vi "uTTA_Calibration_VOffs.vi"(6 "AR488_in":refnum<visa-resource-name>, 7 "CommandQueue":refnum<queue>, 8 "error in":errorcluster, 9 "FunctionGen":refnum<visa-resource-name>, 10 "DataQueue":refnum<queue>, 11 "FDMS_FileIn":refnum<k34>) -> (0 "error out":errorcluster, 1 "FunctionGen_out":refnum<visa-resource-name>, 2 "abort":bool, 3 "FDMS_FileOut":refnum<k34>, 4 "AR488_out":refnum<visa-resource-name>)   [LabVIEW 2021]
uses:
  <vilib>/Utility/miscctls.llb/LVPointTypeDef.ctl
  <vilib>/Analysis/6fits.llb/Curve Fitting Criteria.ctl
  98f5d860-8e0d-4648-8282-1f02ee17b982.vi
  <vilib>/Analysis/NI_AALPro.lvlib
panel:
  out "Channel":i32
  out "VOFF Cal.":T1(graph)
  out "VOFF DAC slope":dbl format="%#_4pV/Digit"
  out "VOFF DAC Residue":dbl caption="Residue" format="%.3p"
  out "VOFF DAC Offset":dbl format="%#_6pV"
  out "ADC_Values":dbl[](array[numeric]) format="%#.2g"
  out "ADC_Variance":dbl[](array[numeric]) format="%#.2g"
  in  "Start DAC VOFF":bool
  in  "VOFF DAC Inc":i32=1000 caption="DAC Incements" min=0 max=32767 step=1 format="%d Counts/Step"
  out "Status":string="Exit"
  in  "stop":bool
  # "1. Connect the DMM in voltage measurement mode between the TP323.x and Ground \n2. Connect a ground lead to the outer Conductor of the BNC line to provide propper grounding\n3. Start the calibration"
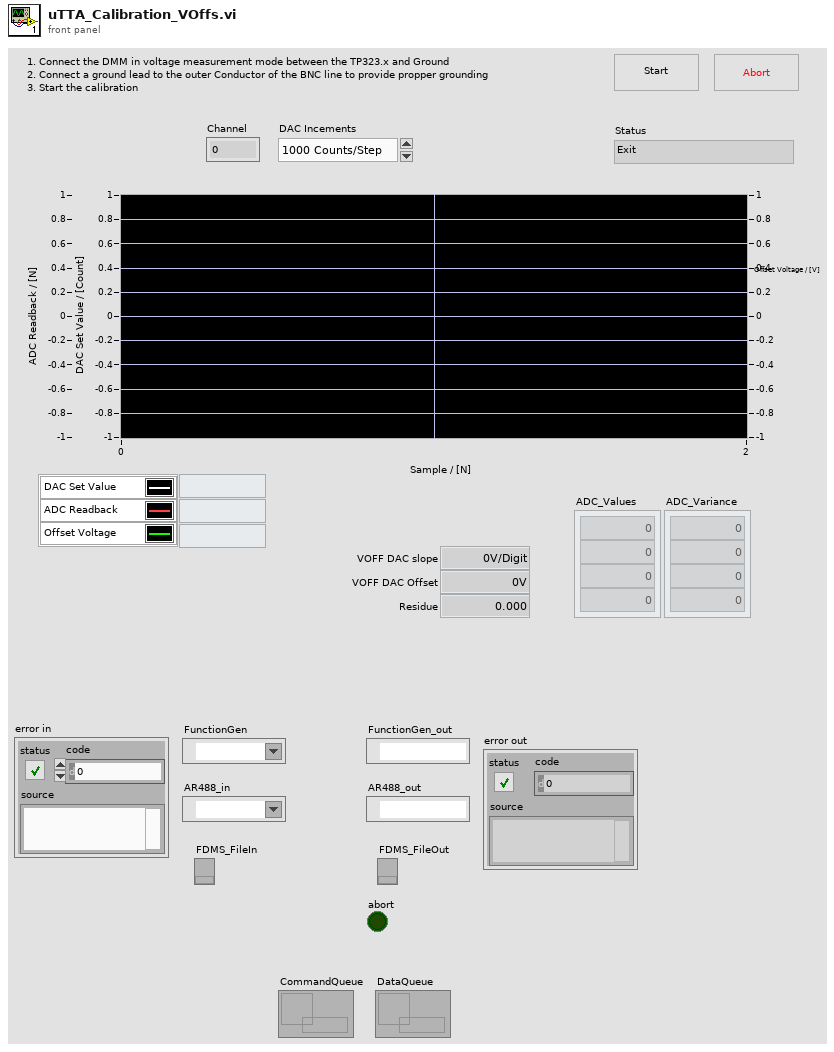
[diagram p1: front panel]
types:
  T1 = cluster{"Ref_Voltage":dbl, "mean":dbl, "mean":dbl}
  T2 = typedef "LVPointTypeDef.ctl" = cluster{"Horizontal":i16, "Vertical":i16}
  T3 = cluster{"Ref_Voltage":dbl, "mean":dbl, "mean":dbl}[]
  T4 = typedef "NI_AALPro.lvlib/Curve Fitting Criteria.ctl" = u16
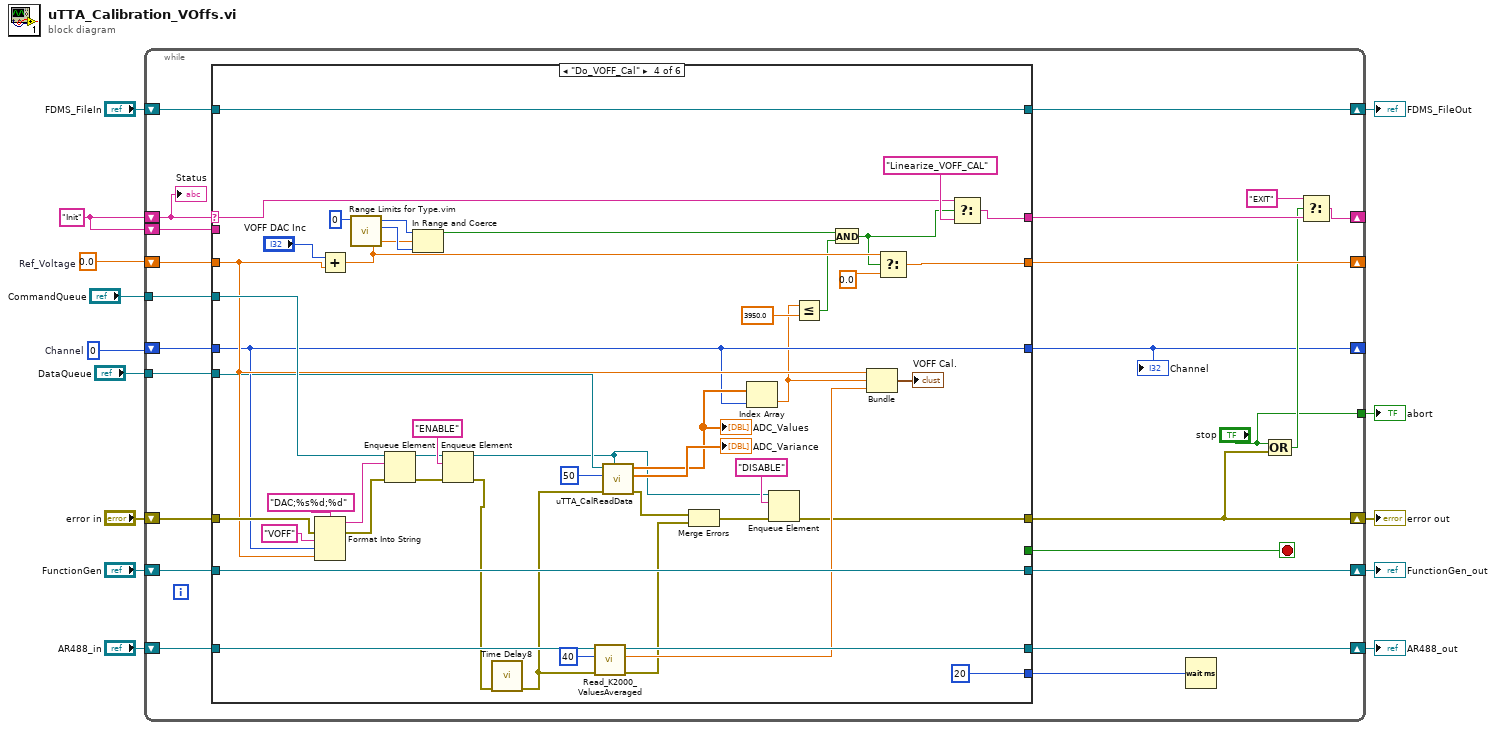
[diagram p0: block diagram]
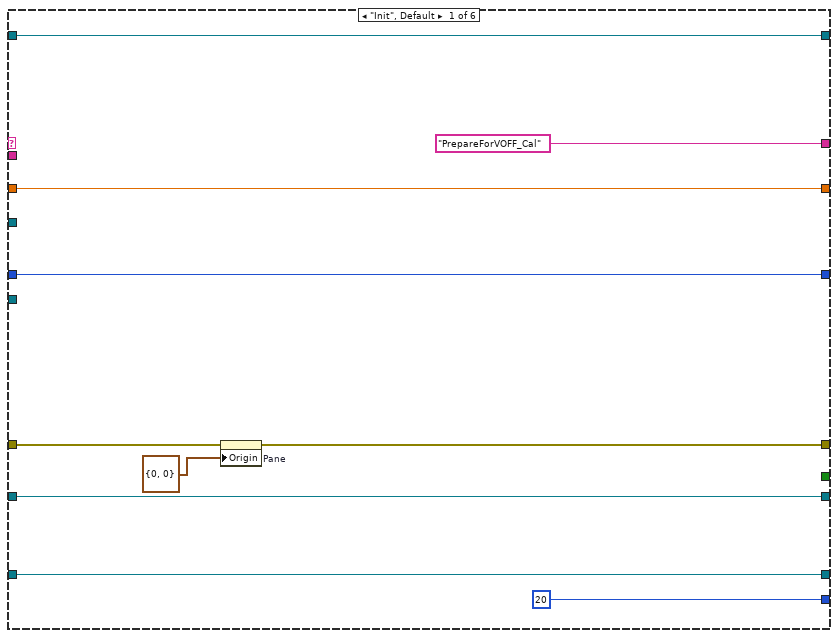
[diagram p2: hidden frame]
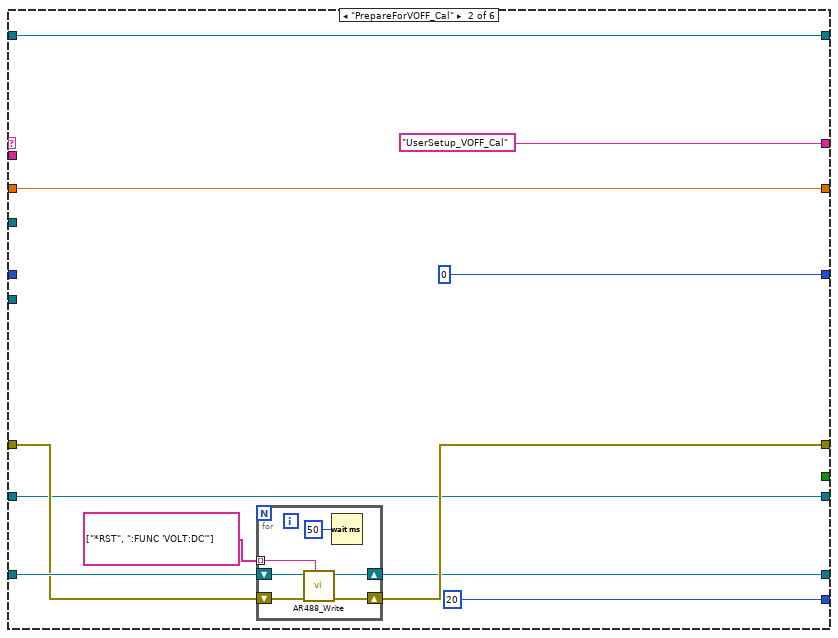
[diagram p3: hidden frame]
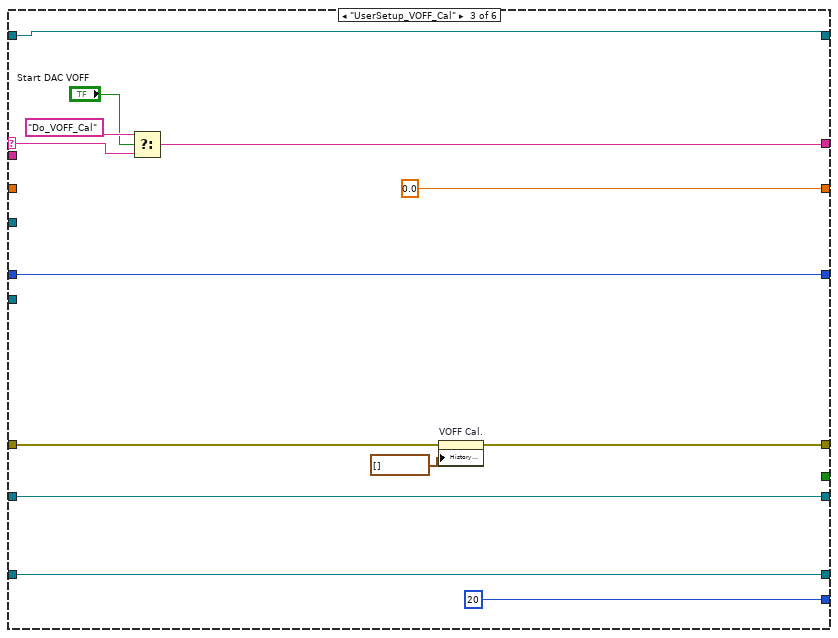
[diagram p4: hidden frame]
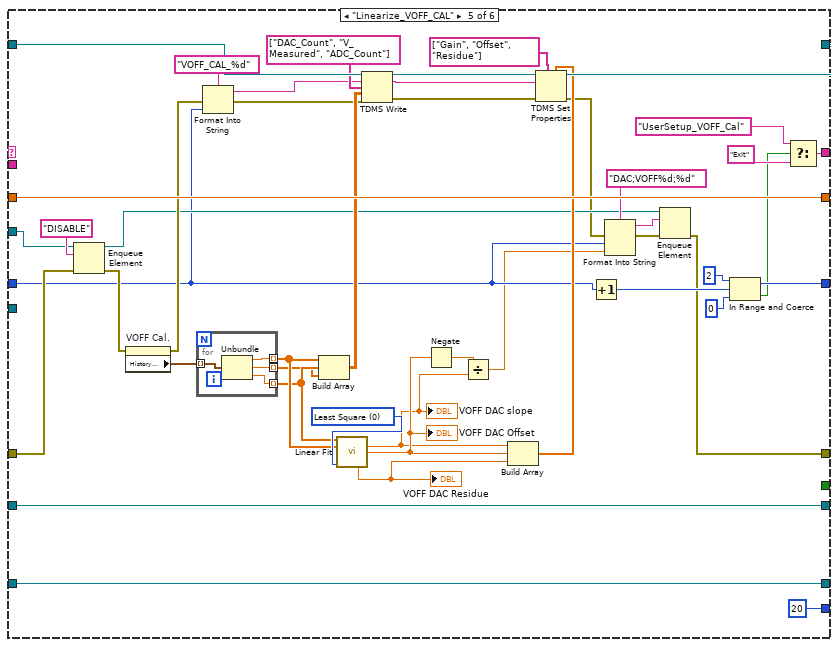
[diagram p5: hidden frame]
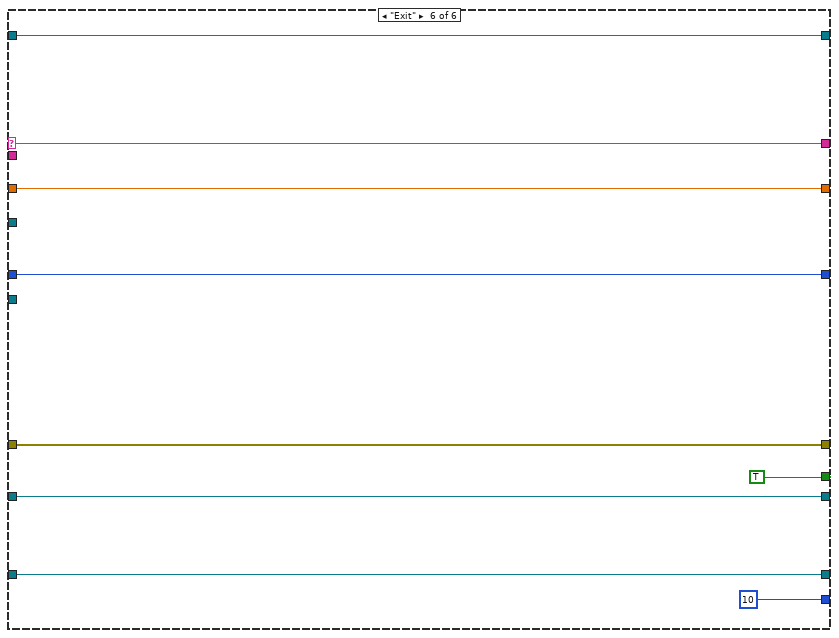
[diagram p6: hidden frame]
diagram:
  w12 = 0  # Channel
  w14 = 0.0  # Ref_Voltage
  w13 = "Init"
  n1 = while {
    shift-right: [w24] -> _
    shift-left: w13 -> [w35]
    shift-right: [w22] -> w7
    shift-left: "error in" -> [w37]
    shift-right: [w33] -> w8
    shift-left: "FunctionGen" -> [w34]
    shift-right: [w32] -> w9
    shift-left: "AR488_in" -> [w31]
    shift-left: w13 -> [w30]
    tunnel: "CommandQueue" -> [w29]
    tunnel: "DataQueue" -> [w28]
    shift-right: [w26] -> _
    shift-left: w14 -> [w27]
    shift-right: [w19] -> w2
    shift-left: "FDMS_FileIn" -> [w18]
    shift-right: [w16] -> _
    shift-left: w12 -> [w17]
    tunnel: ["stop"] -> w1
    stop <- w20 stop-if-true
    n2 = case shown="\"Do_VOFF_Cal\"" w35 {
      selector: w35 -> [_ _ w70 w102 _ w182]
      tunnel: [_ _ _ _ _ TRUE] -> w20
      tunnel: w37 -> [w44 w50 w66 w117 w137 w176]
      tunnel: ["PrepareForVOFF_Cal" ("t") "UserSetup_VOFF_Cal" ("t") w69 w105 w161 w182] -> w25
      tunnel: [w40 w54 w65 w78 w125 w176] -> w22
      tunnel: [u32 20 u32 20 u32 20 u32 20 u32 20 u32 10] -> w36
      tunnel: w34 -> [w43 w49 w77 w123 w169 w175]
      tunnel: [w43 w49 w77 w123 w169 w175] -> w33
      tunnel: [w42 w53 w76 w107 w168 w174] -> w32
      tunnel: w31 -> [w42 w52 w76 w106 w168 w174]
      tunnel: w30 -> [_ _ _ _ _ _]
      tunnel: w29 -> [_ _ _ w121 w138 _]
      tunnel: w28 -> [_ _ _ w93 _ _]
      tunnel: w27 -> [w41 w57 _ w99 w167 w178]
      tunnel: [w41 w57 0.0 w111 w167 w178] -> w26
      tunnel: [w39 w51 w72 w122 w152 w179] -> w19
      tunnel: w18 -> [w39 w51 w72 w122 w151 w179]
      tunnel: w17 -> [w38 _ w71 w95 w128 w177]
      tunnel: [w38 0 ("Channel") w71 w95 w162 w177] -> w16
      frame "Init", Default {
        n3 = property on="Pane" class="Pane"(error in=w44, "Origin"=T2 {"Horizontal"=0, "Vertical"=0}) -> (error out=w40:errorcluster)  [unwired: 1 in, 1 out]
      }
      frame "PrepareForVOFF_Cal" {
        n4 = for {
          tunnel: string[] ["*RST", ":FUNC 'VOLT:DC'"] -> [w63] mode=indexing
          shift-right: [w61] -> w53
          shift-left: w52 -> [w64]
          shift-right: [w60] -> w54
          shift-left: w50 -> [w62]
          n5 = call "AR488_Write.vi"("write"=w63, "error in (no error)"=w62, "VISA Refnum in"=w64) -> ("error out"=w60:errorcluster, "VISA Refnum out"=w61:refnum<visa-resource-name>)  [unwired: 7 in]
          n6 = Wait (ms)(milliseconds to wait=u32 50) -> ()  [unwired: 1 out]
        }
      }
      frame "UserSetup_VOFF_Cal" {
        n7 = Select(t="Do_VOFF_Cal", s="Start DAC VOFF", f=w70) -> (s? t:f=w69:string)
        n8 = property on="VOFF Cal." class="WFChart (strict)"(error in=w66, "History Data"=T3 []) -> (error out=w65:errorcluster)  [unwired: 1 in, 1 out]
      }
      frame "Do_VOFF_Cal" {
        n9 = Format Into String(format string="DAC;%s%d;%d" ("element"), error in=w117, "VOFF" ("input 1"), w95, w99) -> (resulting string=w119:string, error out=w116:errorcluster)  [unwired: 1 in]
        n10 = Add(x="VOFF DAC Inc", y=w99) -> (x+y=w101:dbl)
        n11 = call "Range Limits for Type.vim"("type"=u16 0) -> ("minimum value for type"=w113:u16, "maximum value for type"=w112:u16)  [unwired: 9 in]
        n12 = Enqueue Element(queue=w121, element=w119, error in (no error)=w116) -> (queue out=w82:refnum<queue>, error out=w84:errorcluster)  [unwired: 1 in, 1 out]
        n13 = In Range and Coerce(upper limit=w112, x=w101, lower limit=w113) -> (In Range?=w110:bool)  [unwired: 1 out]
        n14 = Enqueue Element(queue=w82, element="ENABLE", error in (no error)=w84) -> (queue out=w80:refnum<queue>, error out=w83:errorcluster)  [unwired: 1 in, 1 out]
        n15 = call "Time Delay8"("error in (no error)"=w83) -> ("error out"=w94:errorcluster)  [unwired: 10 in]
        n16 = call "Read_K2000_ValuesAveraged.vi"("error in"=w94, "No. Averaged Values"=40, "VISA Refnum in"=w106) -> ("error out"=w90:errorcluster, "mean"=w92:dbl, "VISA Refnum out"=w107:refnum<visa-resource-name>)  [unwired: 6 in]
        n17 = call "uTTA_CalReadData.vi"("Control Queue"=w80, "error in"=w94, "Averaged Values"=50, "Data Queue in"=w93) -> ("error out"=w91:errorcluster, "ADC_Variance"=→"ADC_Variance":dbl[], "ADC_Values"=w96:dbl[])  [unwired: 3 in, 2 out]
        "ADC_Values" <- w96
        n18 = Merge Errors(w91, w90) -> (w79:errorcluster)
        n19 = Index Array(array=w96, index=w95) -> (element=w88:dbl)
        n20 = Enqueue Element(queue=w80, element="DISABLE", error in (no error)=w79) -> (error out=w78:errorcluster)  [unwired: 1 in, 2 out]
        n21 = Less Or Equal?(x=w88, y=3950.0) -> (x <= y?=w86:bool)
        n22 = And(x=w110, y=w86) -> (x .and. y?=w87:bool)
        n23 = Bundle("Ref_Voltage"=w99, "mean"=w88, "mean"=w92) -> (→"VOFF Cal.":T1)  [unwired: 1 in]
        n24 = Select(t=w101, s=w87, f=0.0 ("t")) -> (s? t:f=w111:dbl)
        n25 = Select(t=w102, s=w87, f="Linearize_VOFF_CAL" ("t")) -> (s? t:f=w105:string)
      }
      frame "Linearize_VOFF_CAL" {
        w157 = T4 0 items=["Least Square", "Least Absolute Residual", "Bisquare"] ("method")
        n26 = Enqueue Element(queue=w138, element="DISABLE", error in (no error)=w137) -> (queue out=w129:refnum<queue>, error out=w136:errorcluster)  [unwired: 1 in, 1 out]
        n27 = property on="VOFF Cal." class="WFChart (strict)"(error in=w136) -> (error out=w141:errorcluster, "History Data"=w156:T3)  [unwired: 1 in, 1 out]
        n28 = for {
          tunnel: w156 -> [w173] mode=indexing
          tunnel: [w171] -> w149 mode=indexing
          tunnel: [w172] -> w150 mode=indexing
          tunnel: [w170] -> w124 mode=indexing
          n29 = Unbundle(w173) -> ("Ref_Voltage"=w172:dbl, "mean"=w170:dbl, "mean"=w171:dbl)
        }
        n30 = Format Into String(format string="VOFF_CAL_%d", error in=w141, w128) -> (resulting string=w145:string, error out=w142:errorcluster)  [unwired: 1 in]
        n31 = Build Array(w150, w149, w124) -> (w148:dbl[][])
        n32 = call <vilib>:"Linear Fit.vi"("Y"=w149, "X"=w150, "method"=w157) -> ("slope"=w133:dbl, "intercept"=w135:dbl, "residue"=w158:dbl)  [unwired: 8 in, 2 out]
        "VOFF DAC Offset" <- w135
        "VOFF DAC Residue" <- w158
        "VOFF DAC slope" <- w133
        n33 = TDMS Write(0:w151, 5:w145, 7:string[] ["DAC_Count", "V_Measured", "ADC_Count"], 9:w148, 11:w142) -> (4:w155:refnum<k34>, 6:w144:string, 15:w154:errorcluster)  [unwired: 1 in, 1 out]
        n34 = Negate(x=w135) -> (-x=w134:dbl)
        n35 = Divide(x=w134, y=w133) -> (x/y=w127:dbl)
        n36 = Build Array(w133, w135, w158) -> (w143:dbl[])
        n37 = TDMS Set Properties(5:w143, 7:string[] ["Gain", "Offset", "Residue"] ("property names"), 8:w154, 10:w144, 11:w155) -> (0:w126:errorcluster, 3:w152:refnum<k34>)  [unwired: 1 in, 2 out]
        n38 = Increment(x=w128) -> (x+1=w163:i32)
        n39 = Format Into String(format string="DAC;VOFF%d;%d" ("element"), error in=w126, w128, w127) -> (resulting string=w131:string, error out=w130:errorcluster)  [unwired: 1 in]
        n40 = Enqueue Element(queue=w129, element=w131, error in (no error)=w130) -> (error out=w125:errorcluster)  [unwired: 1 in, 2 out]
        n41 = In Range and Coerce(upper limit=2, x=w163, lower limit=0) -> (coerced(x)=w162:i32, In Range?=w140:bool)
        n42 = Select(t="UserSetup_VOFF_Cal", s=w140, f="Exit") -> (s? t:f=w161:string)
      }
      frame "Exit" {
      }
    }
    "Channel" <- w16
    n43 = Wait (ms)(milliseconds to wait=w36) -> ()  [unwired: 1 out]
    n44 = Compound Arithmetic op=OR("stop", w22) -> (w21:bool)
    n45 = Select(t="EXIT", s=w21, f=w25) -> (s? t:f=w24:string)
    "Status" <- w35
  }
  "AR488_out" <- w9
  "FunctionGen_out" <- w8
  "error out" <- w7
  "FDMS_FileOut" <- w2
  "abort" <- w1
